vi "dfd_MRate Check Aliasing.vi"(6 "filtering mode":T1=2 items=["No Rate Change", "Interpolation", "Decimation"], 7 "order":i32=4, 8 "error in":errorcluster, 9 "fs in [Hz]":dbl=1000.0, 10 "freq specs":T2={"fpass"=55.0, "fstop"=70.0}, 11 "factor":i32=4) -> (0 "error out":errorcluster, 1 "filter fs [Hz]":dbl=1000.0, 2 "dup freq specs":T2={"fpass"=55.0, "fstop"=70.0}, 3 "dup factor":i32=4, 5 "dup order":i32=4)   [LabVIEW 2017, in "NI_DigFilterLicensed.lvlib"]
uses:
  <vilib>/addons/Digital Filter Design/NI_DigFilterLicensed.lvlib
  <vilib>/addons/Digital Filter Design/_Objects.llb/DFD Multirate Filter Specification (Design).ctl
  <vilib>/addons/Digital Filter Design/_Objects.llb/DFD Multirate Filtering Mode.ctl
  <vilib>/addons/Digital Filter Design/_Misc.llb/dfd_Error Handlers (Multiple).vi
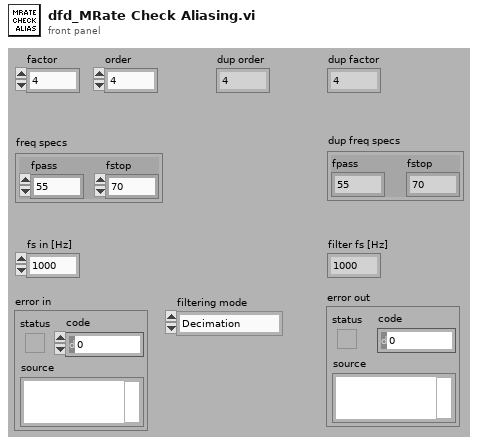
[diagram p1: front panel]
types:
  T1 = typedef "NI_DigFilterLicensed.lvlib/DFD Multirate Filtering Mode.ctl" = u16
  T2 = typedef "NI_DigFilterLicensed.lvlib/DFD Multirate Filter Specification (Design).ctl" = cluster{"fpass":dbl, "fstop":dbl}
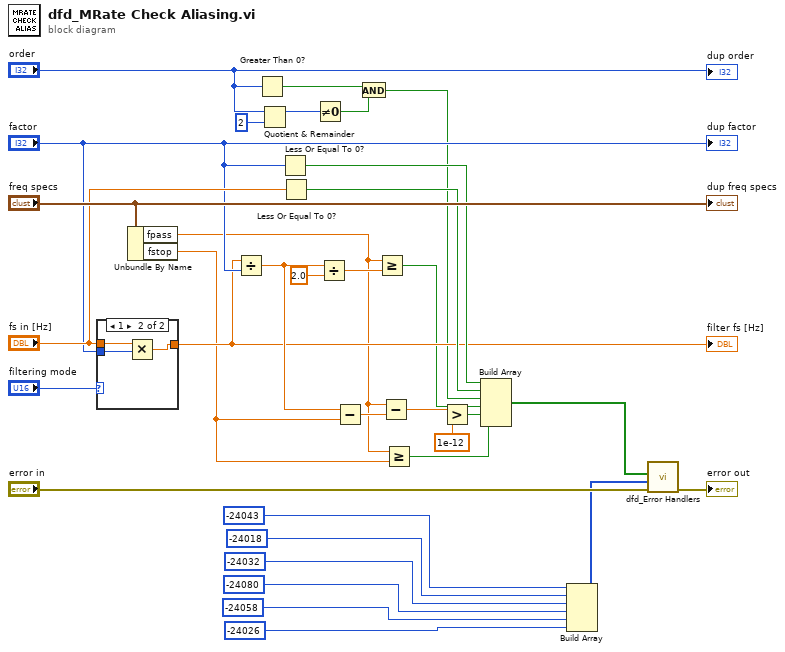
[diagram p0: block diagram]
diagram:
  n1 = case shown="1" "filtering mode" {
    tunnel: "fs in [Hz]" -> [w35 w38]
    tunnel: "factor" -> [_ w37]
    tunnel: [w35 w36] -> w10
    frame 0, Default {
    }
    frame 1 {
      n2 = Multiply(x=w38, y=w37) -> (x*y=w36:dbl)
    }
  }
  "filter fs [Hz]" <- w10
  n3 = Unbundle By Name("freq specs") -> ("fpass"=w9:dbl, "fstop"=w4:dbl)
  n4 = Divide(x=w10, y="factor") -> (x/y=w18:dbl)
  n5 = Greater Than 0?(x="order") -> (x > 0?=w26:bool)
  n6 = Quotient & Remainder(x="order", y=2) -> (x-y*floor(x/y)=w27:i32)  [unwired: 1 out]
  n7 = Less Or Equal To 0?(x="factor") -> (x <= 0?=w15:bool)
  n8 = Less Or Equal To 0?(x="fs in [Hz]") -> (x <= 0?=w14:bool)
  n9 = Not Equal To 0?(x=w27) -> (x != 0?=w13:bool)
  n10 = Divide(x=w18, y=2.0) -> (x/y=w16:dbl)
  n11 = Subtract(x=w18, y=w4) -> (x-y=w31:dbl)
  n12 = And(x=w26, y=w13) -> (x .and. y?=w8:bool)
  n13 = Greater Or Equal?(x=w9, y=w16) -> (x >= y?=w7:bool)
  n14 = Subtract(x=w9, y=w31) -> (x-y=w30:dbl)
  n15 = Greater Or Equal?(x=w9, y=w4) -> (x >= y?=w20:bool)
  n16 = Greater?(x=w30, y=1e-12) -> (0:w32:bool)
  n17 = Build Array(w15, w14, w8, w7, w32, w20) -> (w24:bool[])
  n18 = Build Array(-24043 ("ERR_FACTOR_LE_ZERO"), -24018 ("ERR_FS_LE_ZERO"), -24032 ("ERR_ORDER_ODD"), -24080 ("ERR_FPASS_TOO_HIGH"), -24058 ("ERR_FSTOP_TOO_HIGH"), -24026 ("ERR_FREQ_SEQ_WRONG")) -> (w25:i32[])
  n19 = call-poly <vilib>:"dfd_Error Handlers.vi"("error in (no error)"="error in", "error sources"=w25, "condition failed?"=w24) -> ("error out"=→"error out":errorcluster)  [unwired: 8 out]
  "dup factor" <- "factor"
  "dup order" <- "order"
  "dup freq specs" <- "freq specs"
